vi "AddUser.vi"() -> (0 "drop?":bool=TRUE, 1 "Authority 2":string(combo), 2 "Password 2":string, 3 "Username 2":string)   [LabVIEW 2015]
panel:
  in  "Authority":string(combo)="GENERAL"
  in  "Cancel":bool
  in  "Username":string
  in  "Password":string
  in  "OK":bool
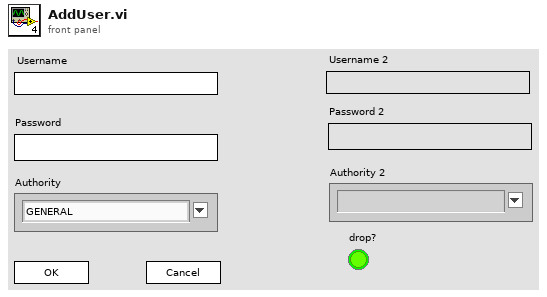
[diagram p1: front panel]
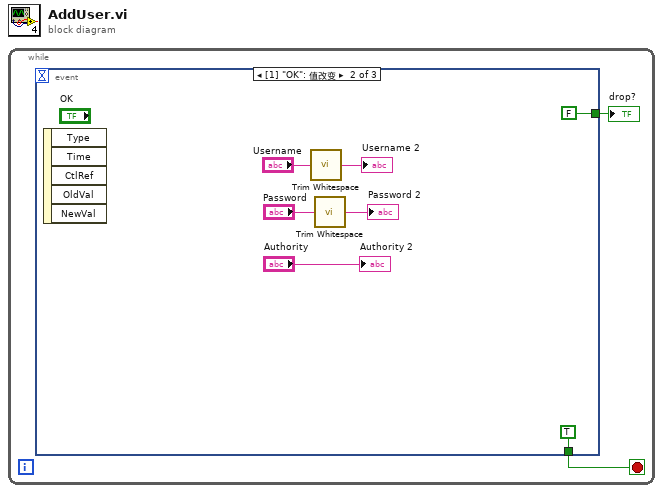
[diagram p0: block diagram]
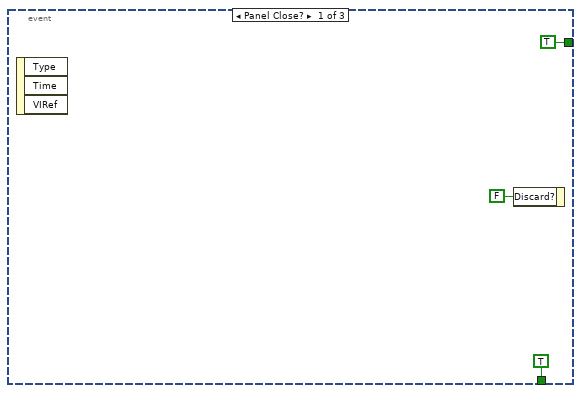
[diagram p2: hidden frame]
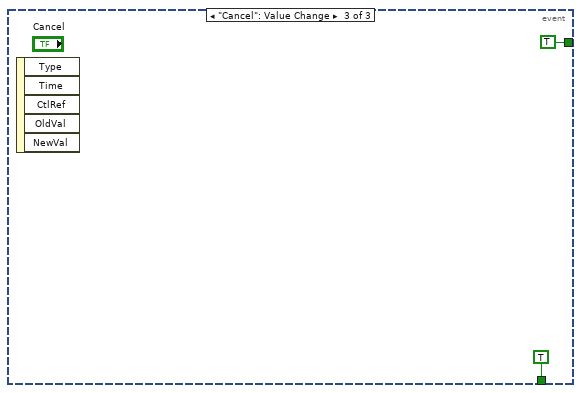
[diagram p3: hidden frame]
diagram:
  n1 = while {
    stop <- w1 stop-if-true
    n2 = event shown="[1] \"OK\": 值改变" {
      selector: _ -> [_ _ _]
      dyn-events: _ -> [_ _ _]
      timeout: _ -> [_ _ _]
      tunnel: [TRUE FALSE TRUE] -> w2
      tunnel: [TRUE TRUE TRUE] -> w1
      event Panel Close? {
        n3 = event-data() -> ()  [unwired: 1 in, 3 out]
        n4 = event-data("Discard?"=FALSE ("放弃？")) -> ()  [unwired: 1 in, 1 out]
      }
      event "OK": Value Change {
        n5 = event-data() -> ()  [unwired: 1 in, 5 out]
        n6 = call <vilib>:"Trim Whitespace.vi"("string"="Username") -> ("trimmed string"=→"Username 2":string)  [unwired: 1 in]
        n7 = call <vilib>:"Trim Whitespace.vi"("string"="Password") -> ("trimmed string"=→"Password 2":string)  [unwired: 1 in]
        "Authority 2" <- "Authority"
      }
      event "Cancel": Value Change {
        n8 = event-data() -> ()  [unwired: 1 in, 5 out]
      }
    }
    "drop?" <- w2
  }
